vi "Gen - File Directory.vi"(6 "File Dir":T1=enum."Config", 8 "Error In":errorcluster) -> (0 "error out":errorcluster, 2 "Application:Kind":T2(ring), 3 "Application Directory":path)   [LabVIEW 2020]
uses:
  Control/State - Directory.ctl
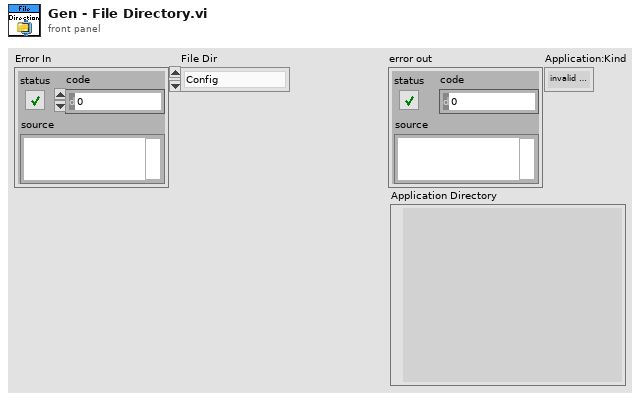
[diagram p1: front panel]
types:
  T1 = typedef "State - Directory.ctl" = enum16{"Plant", "Config", "Admin", "Password", "Modules", "Dialog Box", "SubVI", "Setting"}
  T2 = enum32{"invalid app kind", "Development System", "Run Time System", "Student Edition", "Embedded LabVIEW", "Evaluation", "Custom"}
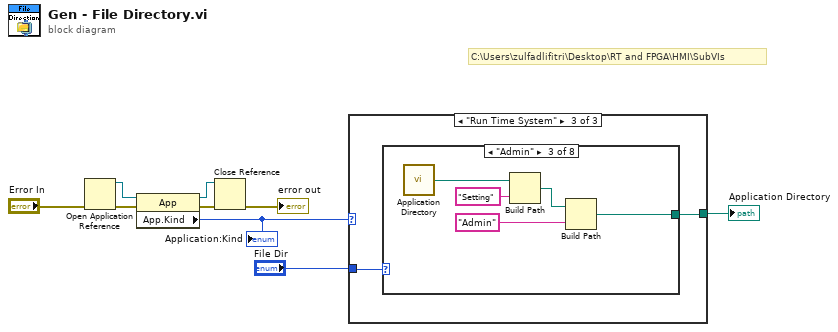
[diagram p0: block diagram]
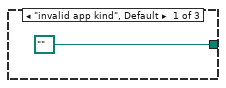
[diagram p2: hidden frame]
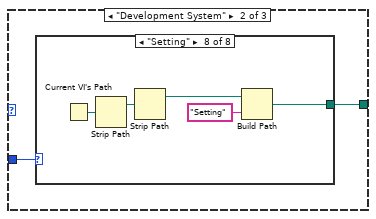
[diagram p3: hidden frame]
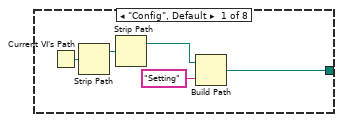
[diagram p4: hidden frame]
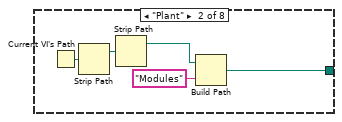
[diagram p5: hidden frame]
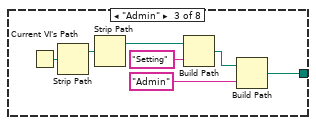
[diagram p6: hidden frame]
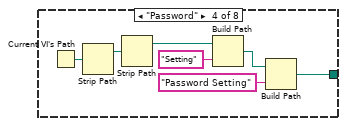
[diagram p7: hidden frame]
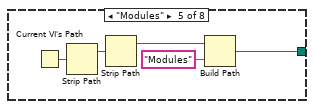
[diagram p8: hidden frame]
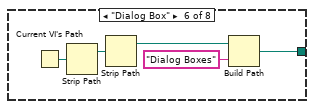
[diagram p9: hidden frame]
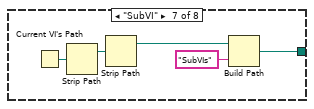
[diagram p10: hidden frame]
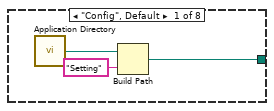
[diagram p11: hidden frame]
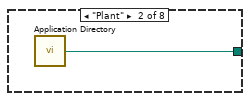
[diagram p12: hidden frame]
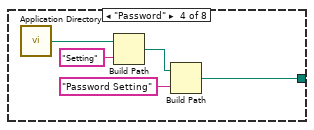
[diagram p13: hidden frame]
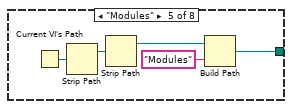
[diagram p14: hidden frame]
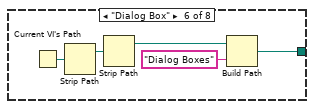
[diagram p15: hidden frame]
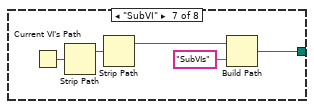
[diagram p16: hidden frame]
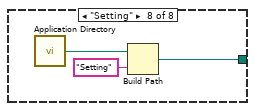
[diagram p17: hidden frame]
diagram:
  # "C:\\Users\\zulfadlifitri\\Desktop\\RT and FPGA\\HMI\\SubVIs"
  n1 = Open Application Reference(8:"Error In") -> (0:w8:errorcluster, 3:w9:refnum<vi>)  [unwired: 3 in]
  n2 = property class="App"(reference=w9, error in=w8) -> (reference out=w6:refnum<vi>, error out=w7:errorcluster, "App.Kind"=w5:T2)
  "Application:Kind" <- w5
  n3 = Close Reference(reference=w6, error in (no error)=w7) -> (error out=→"error out":errorcluster)
  n4 = case shown="\"Run Time System\"" w5 {
    tunnel: [path "" ("Application Directory") w12 w58] -> w1
    tunnel: "File Dir" -> [_ w11 w57]
    frame "invalid app kind", Default {
    }
    frame "Development System" {
      n5 = case shown="\"Setting\"" w11 {
        tunnel: [w13 w18 w23 w31 w37 w42 w47 w52] -> w12
        frame "Config", Default {
          n6 = Current VI's Path() -> (path=w17:path)
          n7 = Strip Path(path=w17) -> (stripped path=w16:path)  [unwired: 1 out]
          n8 = Strip Path(path=w16) -> (stripped path=w15:path)  [unwired: 1 out]
          n9 = Build Path(base path=w15, name or relative path="Setting") -> (appended path=w13:path)
        }
        frame "Plant" {
          n10 = Current VI's Path() -> (path=w22:path)
          n11 = Strip Path(path=w22) -> (stripped path=w21:path)  [unwired: 1 out]
          n12 = Strip Path(path=w21) -> (stripped path=w20:path)  [unwired: 1 out]
          n13 = Build Path(base path=w20, name or relative path="Modules") -> (appended path=w18:path)
        }
        frame "Admin" {
          n14 = Current VI's Path() -> (path=w29:path)
          n15 = Strip Path(path=w29) -> (stripped path=w28:path)  [unwired: 1 out]
          n16 = Strip Path(path=w28) -> (stripped path=w27:path)  [unwired: 1 out]
          n17 = Build Path(base path=w27, name or relative path="Setting") -> (appended path=w24:path)
          n18 = Build Path(base path=w24, name or relative path="Admin") -> (appended path=w23:path)
        }
        frame "Password" {
          n19 = Current VI's Path() -> (path=w36:path)
          n20 = Strip Path(path=w36) -> (stripped path=w35:path)  [unwired: 1 out]
          n21 = Strip Path(path=w35) -> (stripped path=w34:path)  [unwired: 1 out]
          n22 = Build Path(base path=w34, name or relative path="Setting") -> (appended path=w32:path)
          n23 = Build Path(base path=w32, name or relative path="Password Setting") -> (appended path=w31:path)
        }
        frame "Modules" {
          n24 = Current VI's Path() -> (path=w41:path)
          n25 = Strip Path(path=w41) -> (stripped path=w40:path)  [unwired: 1 out]
          n26 = Strip Path(path=w40) -> (stripped path=w39:path)  [unwired: 1 out]
          n27 = Build Path(base path=w39, name or relative path="Modules") -> (appended path=w37:path)
        }
        frame "Dialog Box" {
          n28 = Current VI's Path() -> (path=w46:path)
          n29 = Strip Path(path=w46) -> (stripped path=w45:path)  [unwired: 1 out]
          n30 = Strip Path(path=w45) -> (stripped path=w44:path)  [unwired: 1 out]
          n31 = Build Path(base path=w44, name or relative path="Dialog Boxes") -> (appended path=w42:path)
        }
        frame "SubVI" {
          n32 = Current VI's Path() -> (path=w51:path)
          n33 = Strip Path(path=w51) -> (stripped path=w50:path)  [unwired: 1 out]
          n34 = Strip Path(path=w50) -> (stripped path=w49:path)  [unwired: 1 out]
          n35 = Build Path(base path=w49, name or relative path="SubVIs") -> (appended path=w47:path)
        }
        frame "Setting" {
          n36 = Current VI's Path() -> (path=w56:path)
          n37 = Strip Path(path=w56) -> (stripped path=w55:path)  [unwired: 1 out]
          n38 = Strip Path(path=w55) -> (stripped path=w54:path)  [unwired: 1 out]
          n39 = Build Path(base path=w54, name or relative path="Setting") -> (appended path=w52:path)
        }
      }
    }
    frame "Run Time System" {
      n40 = case shown="\"Admin\"" w57 {
        tunnel: [w60 w62 w63 w69 w73 w78 w83 w88] -> w58
        frame "Config", Default {
          n41 = call <vilib>:"Application Directory.vi"() -> ("Application Directory"=w59:path)
          n42 = Build Path(base path=w59, name or relative path="Setting") -> (appended path=w60:path)
        }
        frame "Plant" {
          n43 = call <vilib>:"Application Directory.vi"() -> ("Application Directory"=w62:path)
        }
        frame "Admin" {
          n44 = call <vilib>:"Application Directory.vi"() -> ("Application Directory"=w66:path)
          n45 = Build Path(base path=w66, name or relative path="Setting") -> (appended path=w64:path)
          n46 = Build Path(base path=w64, name or relative path="Admin") -> (appended path=w63:path)
        }
        frame "Password" {
          n47 = call <vilib>:"Application Directory.vi"() -> ("Application Directory"=w71:path)
          n48 = Build Path(base path=w71, name or relative path="Setting") -> (appended path=w70:path)
          n49 = Build Path(base path=w70, name or relative path="Password Setting") -> (appended path=w69:path)
        }
        frame "Modules" {
          n50 = Current VI's Path() -> (path=w75:path)
          n51 = Strip Path(path=w75) -> (stripped path=w76:path)  [unwired: 1 out]
          n52 = Strip Path(path=w76) -> (stripped path=w77:path)  [unwired: 1 out]
          n53 = Build Path(base path=w77, name or relative path="Modules") -> (appended path=w73:path)
        }
        frame "Dialog Box" {
          n54 = Current VI's Path() -> (path=w80:path)
          n55 = Strip Path(path=w80) -> (stripped path=w81:path)  [unwired: 1 out]
          n56 = Strip Path(path=w81) -> (stripped path=w82:path)  [unwired: 1 out]
          n57 = Build Path(base path=w82, name or relative path="Dialog Boxes") -> (appended path=w78:path)
        }
        frame "SubVI" {
          n58 = Current VI's Path() -> (path=w85:path)
          n59 = Strip Path(path=w85) -> (stripped path=w86:path)  [unwired: 1 out]
          n60 = Strip Path(path=w86) -> (stripped path=w87:path)  [unwired: 1 out]
          n61 = Build Path(base path=w87, name or relative path="SubVIs") -> (appended path=w83:path)
        }
        frame "Setting" {
          n62 = call <vilib>:"Application Directory.vi"() -> ("Application Directory"=w90:path)
          n63 = Build Path(base path=w90, name or relative path="Setting") -> (appended path=w88:path)
        }
      }
    }
  }
  "Application Directory" <- w1
